vi "transDofToUk.vi"(8 "error in (no error)":errorcluster, 10 "State in DOF":dbl[](array[numeric]), 11 "ZTAAC in":refnum<class "ZTAAC.lvclass">) -> (0 "error out":errorcluster, 2 "uk Array":dbl[](array[numeric]), 3 "ZTAAC out":refnum<class "ZTAAC.lvclass">)   [LabVIEW 2016, in "OfcFunc.lvlib" / "ZTAAC.lvclass"]
doc: "Transform the degree of freedom (DOF) to uk based on the index array of DOF."
uses:
  ZTAAC.lvclass
  ZTAAC.lvclass/ZTAAC.ctl
  OptStateEsti/OptStateEsti.lvclass
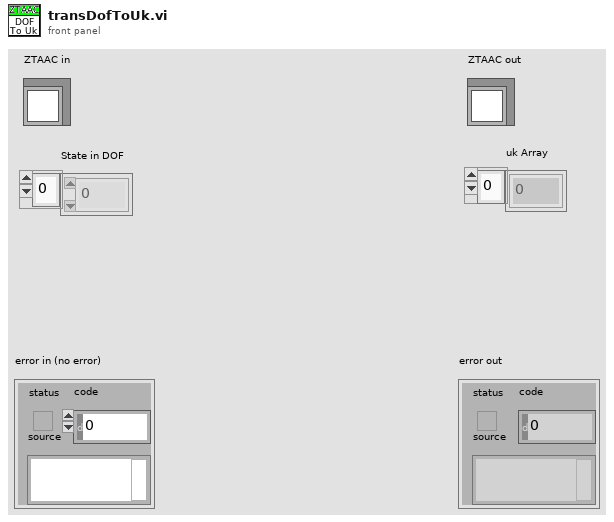
[diagram p1: front panel]
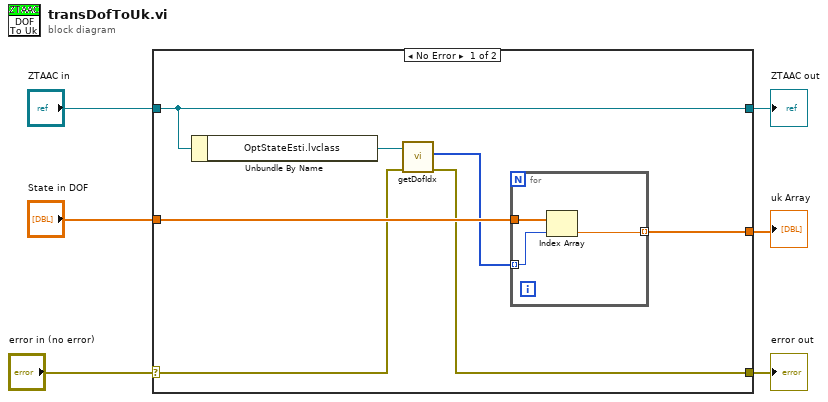
[diagram p0: block diagram]
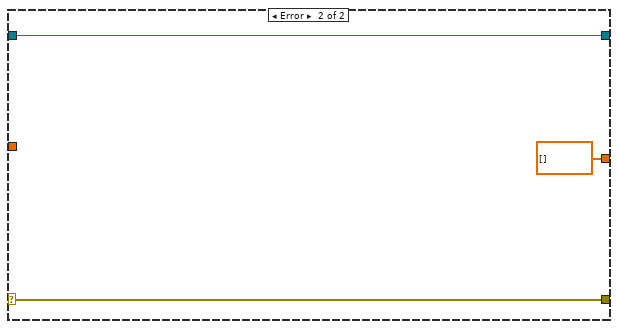
[diagram p2: hidden frame]
diagram:
  n1 = case shown="No Error" "error in (no error)" {
    selector: "error in (no error)" -> [w8 w19]
    tunnel: [w7 w19] -> w5
    tunnel: [w13 w18] -> w3
    tunnel: "ZTAAC in" -> [w13 w18]
    tunnel: "State in DOF" -> [w11 _]
    tunnel: [w9 dbl[] []] -> w1
    frame No Error {
      n2 = Unbundle By Name(w13) -> ("OptStateEsti.lvclass"=w12:refnum<class "OptStateEsti.lvclass">)
      n3 = call "getDofIdx.vi"("error in (no error)"=w8, "OptStateEsti in"=w12) -> ("error out"=w7:errorcluster, "dofIdx"=w10:i32[])  [unwired: 7 in, 1 out]
      n4 = for {
        tunnel: w11 -> [w16]
        tunnel: w10 -> [w15] mode=indexing
        tunnel: [w14] -> w9 mode=indexing
        n5 = Index Array(array=w16, index=w15) -> (element=w14:dbl)
      }
    }
    frame Error {
    }
  }
  "error out" <- w5
  "ZTAAC out" <- w3
  "uk Array" <- w1
